vi "ConvertGoop2ToGoop3_SaveAll.vi"(8 "error out 2":errorcluster, 11 "Cluster":T6) -> (0 "error out":errorcluster)   [LabVIEW 2010]
uses:
  ConvertGoop2ToGoop3_ClassInfo.ctl
  LvClass_class/GDSLvCLass_ClassSettingsType.ctl
  LvClass_class/GDSLvClass_PlugIn.ctl
  LvClass_class/GDSLvClass_PlugInTypes.ctl
  <vilib>/Utility/miscctls.llb/LVPositionTypeDef.ctl
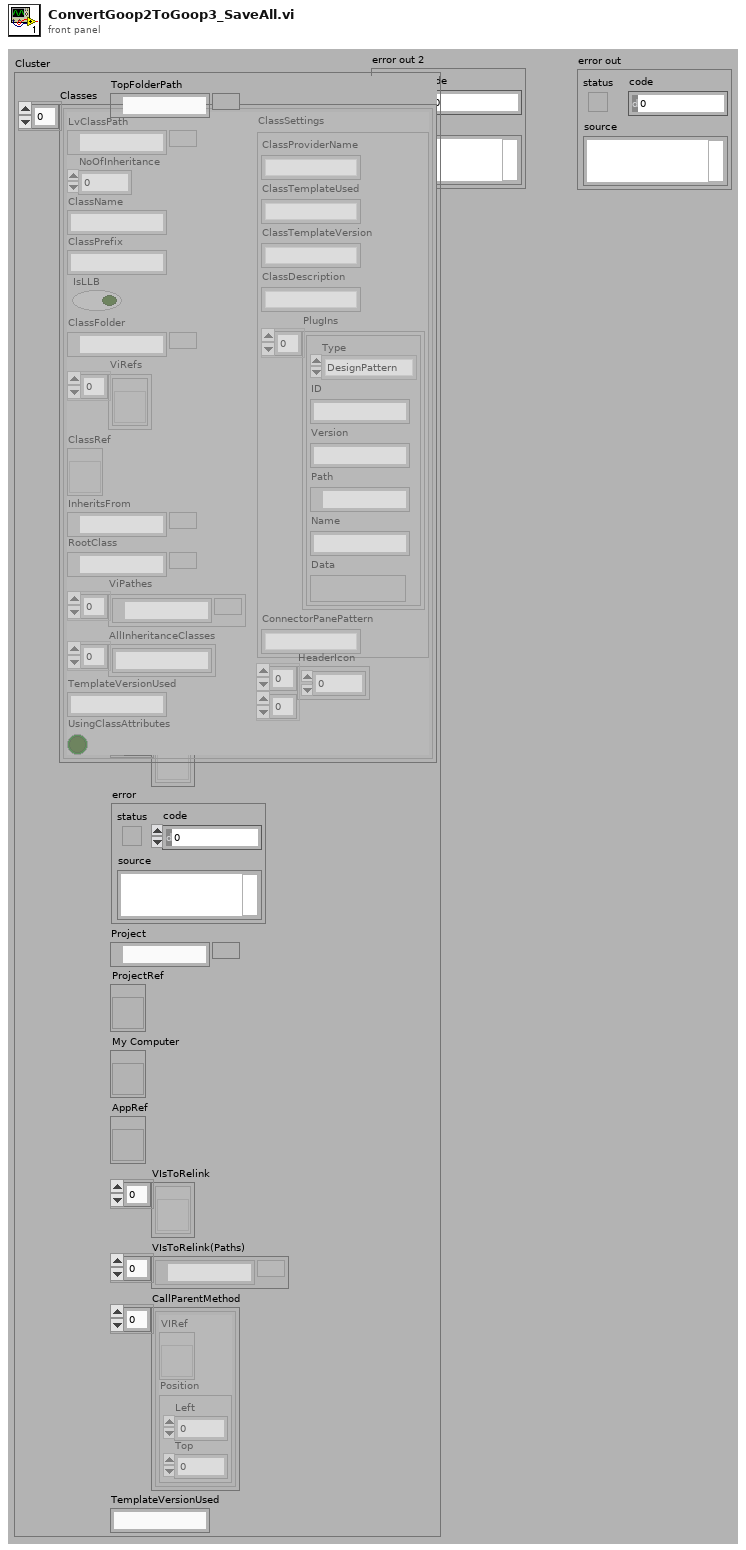
[diagram p1: front panel]
types:
  T1 = typedef "ConvertGoop2ToGoop3_ClassInfo.ctl" = cluster{"NoOfInheritance":i32, "LvClassPath":path, "ClassName":string, "ClassPrefix":string, "IsLLB":bool, "ClassFolder":path, "ViRefs":refnum<vi>[], "ClassRef":refnum<vi>, "InheritsFrom":path, "RootClass":path, "ViPathes":path[], "AllInheritanceClasses":string[], "TemplateVersionUsed":string, "UsingClassAttributes":bool, "ClassSettings":T2, "HeaderIcon":u8[][]}
  T2 = typedef "GDSLvCLass_ClassSettingsType.ctl" = cluster{"ClassProviderName":string, "ClassTemplateUsed":string, "ClassTemplateVersion":string, "ClassDescription":string, "PlugIns":T3[], "ConnectorPanePattern":string}
  T3 = typedef "GDSLvClass_PlugIn.ctl" = cluster{"Type":T4, "ID":string, "Version":string, "Path":path, "Name":string, "Data":variant}
  T4 = typedef "GDSLvClass_PlugInTypes.ctl" = enum16{"DesignPattern", "MethodTypes"}
  T5 = typedef "LVPositionTypeDef.ctl" = cluster{"Left":i32, "Top":i32}
  T6 = cluster{"TopFolderPath":path, "Classes":T1[], "SetToDynamicDispatch":refnum<vi>[], "error":errorcluster, "Project":path, "ProjectRef":refnum<vi>, "My Computer":refnum<vi>, "AppRef":refnum<vi>, "VIsToRelink":refnum<vi>[], "VIsToRelink(Paths)":path[], "CallParentMethod":cluster{"VIRef":refnum<vi>, "Position":T5}[], "TemplateVersionUsed":string}
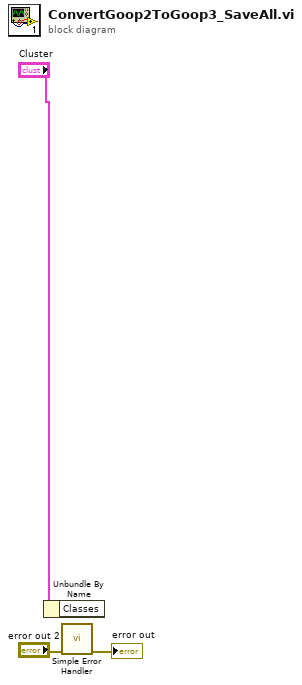
[diagram p0: block diagram]
diagram:
  n1 = Unbundle By Name("Cluster") -> ()  [unwired: 1 out]
  n2 = call <vilib>:"Simple Error Handler.vi"("error in (no error)"="error out 2") -> ("error out"=→"error out":errorcluster)  [unwired: 4 in, 4 out]
